vi "HTS_WELL_#_TO_POS.vi"(4 "Well Number (0-95)":i32 min=0 max=95 step=1) -> (1 "Well Position":T1)   [LabVIEW 2009]
uses:
  HTS_WELL.ctl
  HTS_COLUMN.ctl
  HTS_ROW.ctl
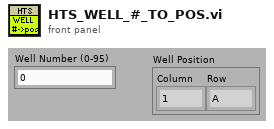
[diagram p1: front panel]
types:
  T1 = typedef "HTS_WELL.ctl" = cluster{"Column":T2, "Row":T3}
  T2 = typedef "HTS_COLUMN.ctl" = enum16{"1", "2", "3", "4", "5", "6", "7", "8", "9", "10", "11", "12"}
  T3 = typedef "HTS_ROW.ctl" = enum16{"A", "B", "C", "D", "E", "F", "G", "H"}
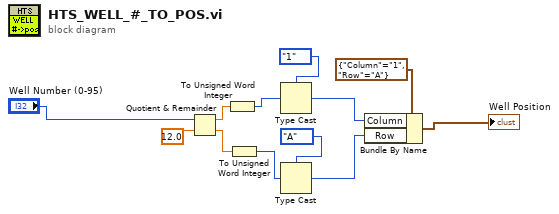
[diagram p0: block diagram]
diagram:
  n1 = Quotient & Remainder(x="Well Number (0-95)", y=12.0) -> (x-y*floor(x/y)=w6:dbl, floor(x/y)=w8:dbl)
  n2 = To Unsigned Word Integer(number=w6) -> (unsigned 16bit integer=w5:u16)
  n3 = To Unsigned Word Integer(number=w8) -> (unsigned 16bit integer=w7:u16)
  n4 = Type Cast(type=HTS_COLUMN."1" ("Column"), x=w5) -> (*(type *) &x=w3:T2)
  n5 = Type Cast(type=HTS_ROW."A" ("Row"), x=w7) -> (*(type *) &x=w2:T3)
  n6 = Bundle By Name(cluster=T1 {"Column"=enum."1", "Row"=enum."A"} ("Well"), "Column"=w3, "Row"=w2) -> (→"Well Position":T1)
